vi "Write Paths.vi"(8 "error in (no error)":errorcluster, 10 "Paths":refnum<class "Path Settings.lvclass">[](array[class]), 11 "Setting Database in":refnum<class "Setting Database.lvclass">) -> (0 "error out":errorcluster, 3 "Setting Database out":refnum<class "Setting Database.lvclass">)   [LabVIEW 2019, in "Setting Database.lvclass"]
uses:
  Setting Database.lvclass
  Path Settings/Path Settings.lvclass
  Setting Database.lvclass/Setting Database.ctl
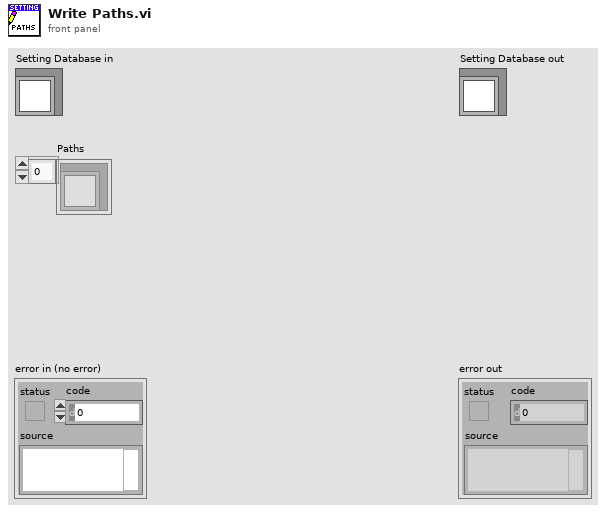
[diagram p1: front panel]
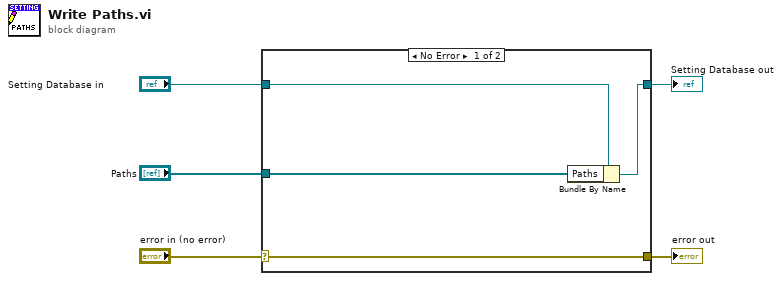
[diagram p0: block diagram]
diagram:
  n1 = case shown="No Error" "error in (no error)" {
    selector: "error in (no error)" -> [w9 w10]
    tunnel: [w9 w10] -> w4
    tunnel: [w7 w11] -> w2
    tunnel: "Setting Database in" -> [w8 w11]
    tunnel: "Paths" -> [w6 _]
    frame No Error {
      n2 = Bundle By Name(cluster=w8, "Paths"=w6) -> (w7:refnum<class "Setting Database.lvclass">)
    }
    frame Error {
    }
  }
  "error out" <- w4
  "Setting Database out" <- w2
